vi "Climber_Determiner.vi"() -> ()   [LabVIEW 2020]
uses:
  Climber_Control_States.ctl
  Globals/Climber_Globals.vi
panel:
  in  "Tune_PIDs":bool
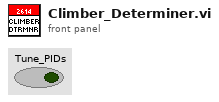
[diagram p1: front panel]
types:
  T1 = typedef "Climber_Control_States.ctl" = enum16{"No-Op", "Manual_%Vbus", "Correct_Outer_Pivot_Offset", "Climbing_Sequence", "Tune_PIDs"}
  T2 = typedef "Climber_Cluster.ctl" = cluster{"Control_State":T1, "Outer_Arm_Pivot_Throttle":dbl, "Outer_Arm_Elevator_Throttle":dbl, "Inner_Arm_Pivot_Throttle":dbl, "Enable_Climber_Sequence":bool}
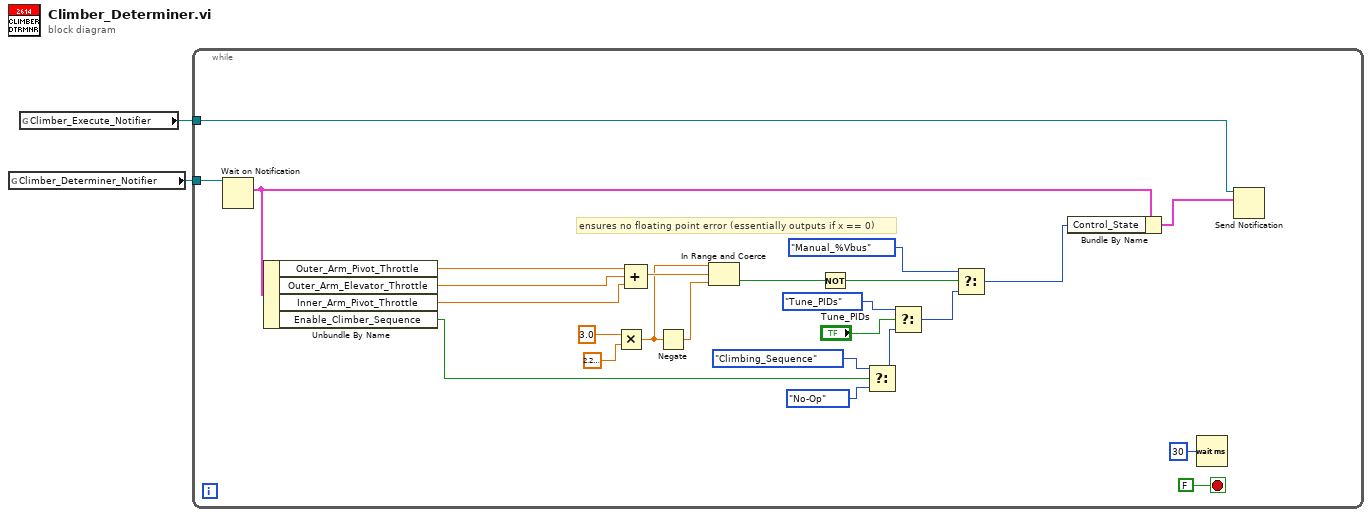
[diagram p0: block diagram]
diagram:
  n1 = global read "Climber_Globals.vi" "Climber_Determiner_Notifier"() -> (w2:refnum<notifier>)
  n2 = global read "Climber_Globals.vi" "Climber_Execute_Notifier"() -> (w1:refnum<notifier>)
  n3 = while {
    tunnel: w2 -> [w27]
    tunnel: w1 -> [w20]
    stop <- FALSE stop-if-true
    # "ensures no floating point error (essentially outputs if x == 0)"
    n4 = Wait on Notification(notifier=w27) -> (notification=w13:T2)  [unwired: 3 in, 3 out]
    n5 = Unbundle By Name(w13) -> ("Outer_Arm_Pivot_Throttle"=w24:dbl, "Outer_Arm_Elevator_Throttle"=w23:dbl, "Inner_Arm_Pivot_Throttle"=w22:dbl, "Enable_Climber_Sequence"=w9:bool)
    n6 = Multiply(x=3.0, y=2.220446049250313e-16) -> (x*y=w10:dbl)
    n7 = Compound Arithmetic op=ADD(w24, w23, w22) -> (w19:dbl)
    n8 = Negate(x=w10) -> (-x=w18:dbl)
    n9 = In Range and Coerce(upper limit=w10, x=w19, lower limit=w18) -> (In Range?=w17:bool)  [unwired: 1 out]
    n10 = Not(x=w17) -> (.not. x?=w8:bool)
    n11 = Select(t=Climber_Control_States."Climbing_Sequence" ("Control_State"), s=w9, f=Climber_Control_States."No-Op" ("Control_State")) -> (s? t:f=w5:T1)
    n12 = Select(t=Climber_Control_States."Tune_PIDs" ("s? t:f"), s="Tune_PIDs", f=w5) -> (s? t:f=w4:T1)
    n13 = Select(t=Climber_Control_States."Manual_%Vbus" ("Control_State"), s=w8, f=w4) -> (s? t:f=w3:T1)
    n14 = Bundle By Name(cluster=w13, "Control_State"=w3) -> (w21:T2)
    n15 = Wait (ms)(milliseconds to wait=u32 30) -> ()  [unwired: 1 out]
    n16 = Send Notification(notification=w21, notifier=w20) -> ()  [unwired: 1 in, 2 out]
  }
